vi "Unflatten.vi"(8 "error in (no error)":errorcluster, 11 "Wavelength iHR320 in":refnum<class "Wavelength ActiveX.lvclass">) -> (0 "error out":errorcluster, 3 "Wavelength iHR320 out":refnum<class "Wavelength ActiveX.lvclass">)   [LabVIEW 2017, in "Wavelength ActiveX.lvclass"]
uses:
  Wavelength ActiveX.lvclass
  Wavelength ActiveX.lvclass/Wavelength ActiveX.ctl
  Global/File Locations.vi
  Scanner/Scanner.lvclass
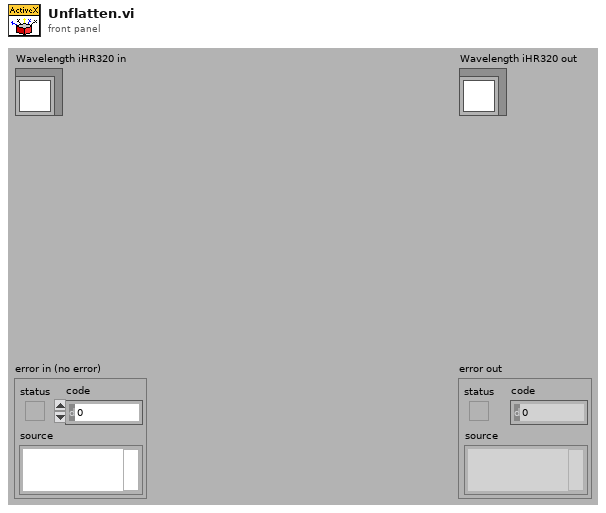
[diagram p1: front panel]
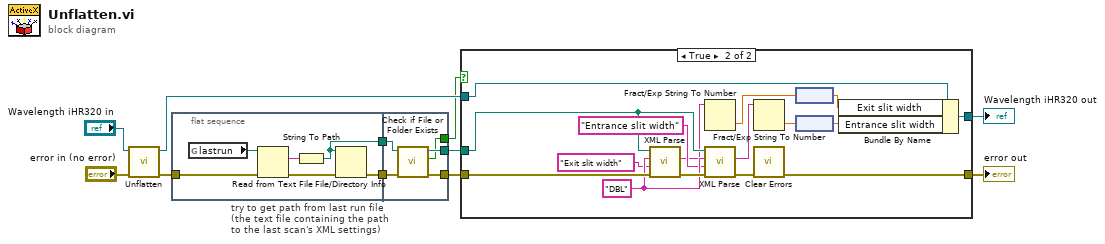
[diagram p0: block diagram]
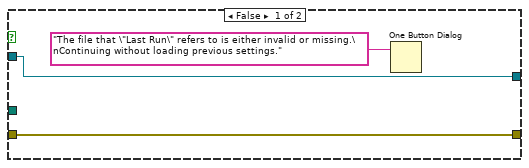
[diagram p2: hidden frame]
diagram:
  n1 = call-parent "Unflatten.vi"("error in (no error)"="error in (no error)", "Scanner in"="Wavelength iHR320 in") -> ("error out"=w7:errorcluster, "Scanner out"=w11:refnum<class "Wavelength ActiveX.lvclass">)  [unwired: 8 in]
  n2 = flat-sequence "try to get path from last run file\n(the text file containing the path\nto the last scan's XML settings)" {
    tunnel: w7 -> [w12]
    tunnel: [w17] -> w3
    tunnel: [w13] -> w2
    tunnel: [w19] -> w6
    tunnel: [w20] -> w5
    tunnel: w3 -> [w22]
    tunnel: w2 -> [w21]
    tunnel: [w18] -> w1
    frame #0 {
      n3 = global read "File Locations.vi" "lastrun"() -> (w15:path)
      n4 = Read from Text File(file (use dialog)=w15, error in=w12) -> (text=w16:string, error out=w14:errorcluster)  [unwired: 4 out]
      n5 = String To Path(string=w16) -> (path=w17:path)
      n6 = File/Directory Info(path=w17, error in=w14) -> (error out=w13:errorcluster)  [unwired: 6 out]
    }
    frame #1 {
      n7 = call <vilib>:"Check if File or Folder Exists.vi"("error in (no error)"=w21, "path"=w22) -> ("error out"=w19:errorcluster, "file or folder exists?"=w18:bool, "dup path"=w20:path)  [unwired: 7 in]
    }
  }
  n8 = case shown="True" w1 {
    tunnel: w11 -> [w25 w41]
    tunnel: [w25 w40] -> w8
    tunnel: w6 -> [w23 w39]
    tunnel: w5 -> [_ w38]
    tunnel: [w23 w26] -> w4
    frame False {
      n9 = One Button Dialog(message="The file that \"Last Run\" refers to is either invalid or missing.\nContinuing without loading previous settings.") -> ()  [unwired: 1 in, 1 out]
    }
    frame True {
      w35 = "DBL"
      n10 = call "XML Parse.vi"("error in (no error)"=w39, "Name String"="Exit slit width", "Type String"=w35, "Path"=w38) -> ("error out"=w37:errorcluster, "String Out"=w29:string)  [unwired: 6 in]
      n11 = Fract/Exp String To Number(string=w29) -> (number=w28:dbl)  [unwired: 3 in, 1 out]
      n12 = call "XML Parse.vi"("error in (no error)"=w37, "Name String"="Entrance slit width", "Type String"=w35, "Path"=w38) -> ("error out"=w36:errorcluster, "String Out"=w32:string)  [unwired: 6 in]
      n13 = Fract/Exp String To Number(string=w32) -> (number=w31:dbl)  [unwired: 3 in, 1 out]
      n14 = call <vilib>:"Clear Errors.vi"("error in (no error)"=w36) -> ("error out"=w26:errorcluster)  [unwired: 5 in, 1 out]
      n15 = node(w28) -> (w27:dbl[unit])
      n16 = node(w31) -> (w30:dbl[unit])
      n17 = Bundle By Name(cluster=w41, "Exit slit width"=w27, "Entrance slit width"=w30) -> (w40:refnum<class "Wavelength ActiveX.lvclass">)
    }
  }
  "error out" <- w4
  "Wavelength iHR320 out" <- w8
